vi "xcorr_packet_FXP.vi"(0 "x":u32, 1 "y":u32, 2 "trigger":bool) -> (8 "out":u64, 9 "valid":bool)   [LabVIEW 2017]
uses:
  <vilib>/rvi/FXPMathLib/basic elements/FxpDiscreteDelay/XNode/nifxpmath_DiscreteDelay.xnode
  <vilib>/rvi/FXPMathLib/FxpAdd/XNode/nifxpmath_Add.xnode
  <vilib>/rvi/FXPMathLib/sim/FxpSim.dll
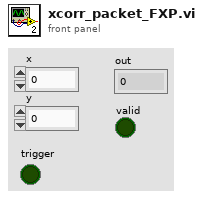
[diagram p1: front panel]
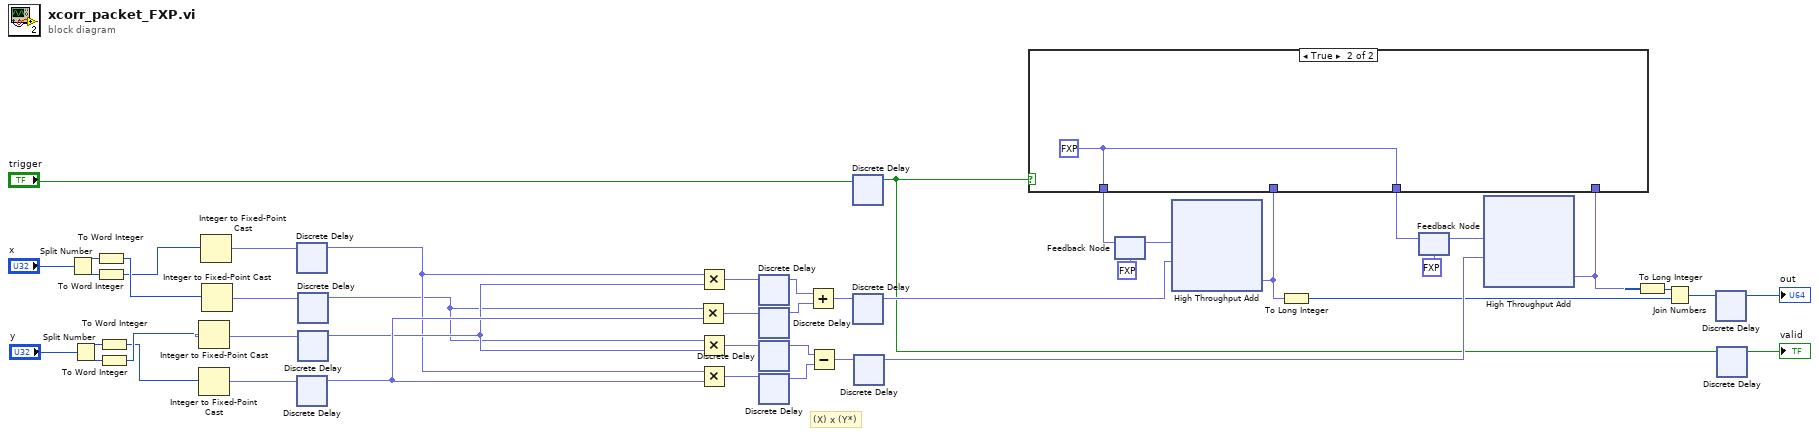
[diagram p0: block diagram]
diagram:
  # "(X) x (Y*)"
  n1 = Split Number(x="x") -> (hi(x)=w38:u16, lo(x)=w39:u16)
  n2 = Split Number(x="y") -> (hi(x)=w40:u16, lo(x)=w41:u16)
  n3 = To Word Integer(number=w38) -> (16bit integer=w18:i16)
  n4 = To Word Integer(number=w39) -> (16bit integer=w17:i16)
  n5 = To Word Integer(number=w40) -> (16bit integer=w15:i16)
  n6 = To Word Integer(number=w41) -> (16bit integer=w16:i16)
  n7 = Integer to Fixed-Point Cast(integer=w16) -> (fixed-point=w25:fxp<+/-,16,1>)  [unwired: 1 in]
  n8 = Integer to Fixed-Point Cast(integer=w15) -> (fixed-point=w27:fxp<+/-,16,1>)  [unwired: 1 in]
  n9 = Integer to Fixed-Point Cast(integer=w17) -> (fixed-point=w23:fxp<+/-,16,1>)  [unwired: 1 in]
  n10 = Integer to Fixed-Point Cast(integer=w18) -> (fixed-point=w24:fxp<+/-,16,1>)  [unwired: 1 in]
  n11 = xnode ("Discrete Delay")("D"=w23) -> ("Q"=w14:fxp<+/-,16,1>)
  n12 = xnode ("Discrete Delay")("D"=w27) -> ("Q"=w26:fxp<+/-,16,1>)
  n13 = xnode ("Discrete Delay")("D"=w24) -> ("Q"=w13:fxp<+/-,16,1>)
  n14 = xnode ("Discrete Delay")("D"=w25) -> ("Q"=w22:fxp<+/-,16,1>)
  n15 = Multiply(x=w13, y=w26) -> (x*y=w33:fxp<+/-,32,1>)
  n16 = Multiply(x=w14, y=w22) -> (x*y=w32:fxp<+/-,32,1>)
  n17 = Multiply(x=w13, y=w22) -> (x*y=w34:fxp<+/-,32,1>)
  n18 = Multiply(x=w14, y=w26) -> (x*y=w35:fxp<+/-,32,1>)
  n19 = xnode ("Discrete Delay")("D"=w32) -> ("Q"=w28:fxp<+/-,32,1>)
  n20 = xnode ("Discrete Delay")("D"=w33) -> ("Q"=w29:fxp<+/-,32,1>)
  n21 = xnode ("Discrete Delay")("D"=w34) -> ("Q"=w30:fxp<+/-,32,1>)
  n22 = xnode ("Discrete Delay")("D"=w35) -> ("Q"=w31:fxp<+/-,32,1>)
  n23 = Add(x=w28, y=w29) -> (x+y=w37:fxp<+/-,32,1>)
  n24 = Subtract(x=w30, y=w31) -> (x-y=w36:fxp<+/-,32,1>)
  n25 = xnode ("Discrete Delay")("D"="trigger") -> ("Q"=w3:bool)
  n26 = xnode ("Discrete Delay")("D"=w37) -> ("Q"=w10:fxp<+/-,32,1>)
  n27 = xnode ("Discrete Delay")("D"=w36) -> ("Q"=w9:fxp<+/-,32,1>)
  n28 = feedback #1(fxp<+/-,64,1> 0.0) -> (w12:fxp<+/-,64,1>)
  n29 = xnode ("High Throughput Add")("x"=w12, "y"=w10) -> ("x+y"=w8:fxp<+/-,64,1>)
  n30 = To Long Integer(number=w8) -> (32bit integer=w7:i32)
  n31 = feedback #2(fxp<+/-,64,1> 0.0) -> (w11:fxp<+/-,64,1>)
  n32 = xnode ("High Throughput Add")("x"=w11, "y"=w9) -> ("x+y"=w1:fxp<+/-,64,1>)
  n33 = case shown="True" w3 {
    tunnel: [w47 w48] -> w20
    tunnel: [w46 w48] -> w19
    tunnel: w8 -> [w46 _]
    tunnel: w1 -> [w47 _]
    frame False {
    }
    frame True {
      w48 = fxp<+/-,64,1> 0.0
    }
  }
  n34 = feedback-in #1(w19) -> ()
  n35 = feedback-in #2(w20) -> ()
  n36 = To Long Integer(number=w1) -> (32bit integer=w6:i32)
  n37 = Join Numbers(hi=w6, lo=w7) -> ((hi.lo)=w5:u64)
  n38 = xnode "Discrete Delay"("D"=w5) -> ("Q"=→"out":u64)
  n39 = xnode "Discrete Delay"("D"=w3) -> ("Q"=→"valid":bool)
